vi "Setup.vi"(8 "Error In":errorcluster, 11 "VI in":refnum<vi>) -> (0 "Error Out":errorcluster, 3 "VI out":refnum<vi>)   [LabVIEW 2017, in "Toolkit.lvlib" / "Tests.lvlib"]
uses:
  Tests.lvlib
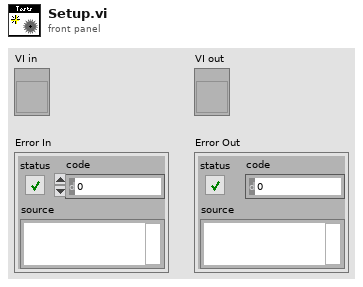
[diagram p1: front panel]
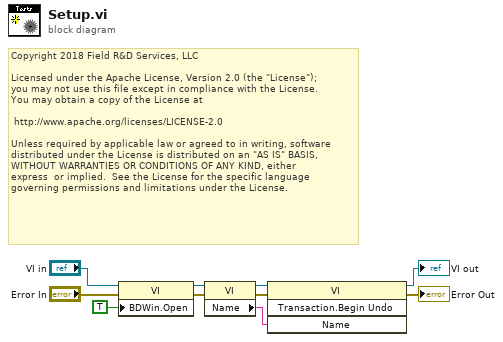
[diagram p0: block diagram]
diagram:
  # "Copyright 2018 Field R&D Services, LLC\n\nLicensed under the Apache License, Version 2.0 (the \"License\");\nyou may not use this file except in compliance with the License.\nYou may obtain a copy of the License at\n\n\thttp://www.apache.org/licenses/LICENSE-2.0\n\nUnless required by applicable law or agreed to in writing, software\ndistributed under the License is distributed on an \"AS IS\" BASIS,\nWITHOUT WARRANTIES OR CONDITIONS OF ANY KIND, either \nexpress  or implied.  See the License for the specific language \ngoverning permissions and limitations under the License."
  n1 = property class="VI"(reference="VI in", error in="Error In", "BDWin.Open"=TRUE ("Block Diagram Window:Open")) -> (reference out=w3:refnum<vi>, error out=w6:errorcluster)
  n2 = property class="VI"(reference=w3, error in=w6) -> (reference out=w5:refnum<vi>, error out=w8:errorcluster, "Name"=w7:string)
  n3 = invoke class="VI" method="Transaction.Begin Undo"(reference=w5, error in=w8, "Name"=w7) -> (reference out=→"VI out":refnum<vi>, error out=→"Error Out":errorcluster)  [unwired: 1 in, 2 out]
